vi "COMI US File Save First.vi"(9 "bIsFromStart":i32, 10 "szFilePath":string, 11 "hDevice":u32) -> (1 "function return":i32, 2 "szFilePath out":string, 3 "hDevice out":u32)   [LabVIEW 2017, in "Comidll.lvlib"]
doc: "int (COMI_US_FileSaveFirst) (HANDLE hDevice, char *szFilePath, int bIsFromStart);"
uses:
  <userlib>/Comidll/Comidll.lvlib
  <userlib>/Comidll/Comidll.dll
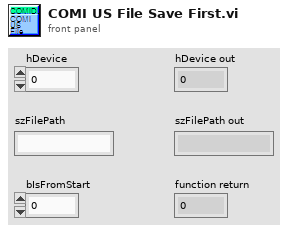
[diagram p1: front panel]
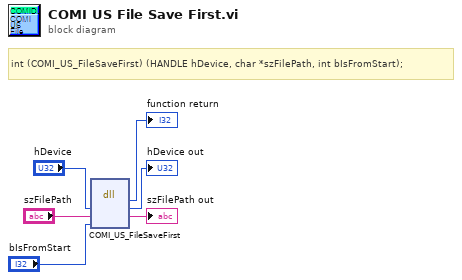
[diagram p0: block diagram]
diagram:
  # "int\t(COMI_US_FileSaveFirst) (HANDLE hDevice, char *szFilePath, int bIsFromStart);"
  n1 = dll-call lib="C:/Program Files/National Instruments/LabVIEW 2017/user.lib/Comidll/Comidll.*" fn="COMI_US_FileSaveFirst"("hDevice"="hDevice", "szFilePath"="szFilePath", "bIsFromStart"="bIsFromStart") -> (→"function return":i32, "hDevice"=→"hDevice out":u32, "szFilePath"=→"szFilePath out":string)  [unwired: 4 in, 2 out]
